vi "Main.vi"(10 "acqpanel":refnum<vi>, 11 "Module Admin":refnum<class "Delacor_lib_QMH_Module Admin.lvclass">) -> ()   [LabVIEW 2019, in "Adquisiion2.lvlib"]
doc: "This template is based off of the Queued Message Handler design pattern and the Queued Message Handler project template that ships with LabVIEW.\n\nThe main difference is that the queue is private to this module and communication between modules is performed via Broadcast and Request events.\n\nRequest events are wrapped in public API methods and are handled in the Event Handling Loop (EHL) of this VI. Any module can register for Broadcast events sent by this module. The EHL generates messages based on user interface actions.\n\nThe Message Handling Loop (MHL) processes messages generated by the EHL, or by other messages. The messages are string values, so new messages can be added easily to the Message Cases case structure in the MHL. Each message cluster can also provide an optional value for Message Data, which is a variant that can be converted to whatever message-specific data is required.\n_____\nBased on Delacor QMH Project Template 5.0.0.82."
uses:
  Adquisiion2.lvlib
  <vilib>/Delacor/Delacor QMH/Libraries/Module Admin_class/Delacor_lib_QMH_Module Admin.lvclass
  Module Data--cluster.ctl
  stop helper loop Argument--cluster.ctl
  <vilib>/Delacor/Delacor QMH/Libraries/Message Queue_class/Delacor_lib_QMH_Message Queue.lvclass/Delacor_lib_QMH_Message Queue.ctl
  Stop Argument--cluster.ctl
  <vilib>/Delacor/Delacor QMH/Libraries/Module Admin_class/Delacor_lib_QMH_Module Admin.lvclass/Delacor_lib_QMH_Module Admin.ctl
  <vilib>/Utility/miscctls.llb/LVPointTypeDef.ctl
  <vilib>/Delacor/Delacor QMH/Libraries/Message Queue_class/Delacor_lib_QMH_Enqueue Message (Single).vi
  <vilib>/Delacor/Delacor QMH/Libraries/Module Admin_class/Delacor_lib_QMH_Get External Launch.vi
  <vilib>/Utility/error.llb/Error Cluster From Error Code.vi
  <vilib>/ErrorRing/Error Ring.xnode
  <vilib>/Delacor/Delacor QMH/Libraries/Message Queue_class/Delacor_lib_QMH_Message Queue.lvclass
panel:
  out "Time Stamp":timestamp
  in  "Simulate MHL Error":bool
  in  "Simulate EHL Error":bool
  out "error out":errorcluster
  out "Status":string
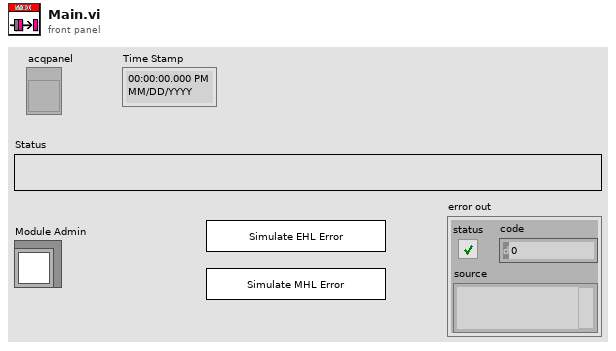
[diagram p1: front panel]
types:
  T1 = typedef "Adquisiion2.lvlib/Request Events--cluster.ctl" = cluster{"Stop Module":refnum<user-event>, "Show Panel":refnum<user-event>, "Hide Panel":refnum<user-event>, "Get Module Execution Status":refnum<user-event>, "Show Diagram":refnum<user-event>, "Start helper loop":refnum<user-event>, "stop helper loop":refnum<user-event>}
  T2 = typedef "Adquisiion2.lvlib/Module Data--cluster.ctl" = cluster{"Status":string}
  T3 = typedef "Adquisiion2.lvlib/stop helper loop Argument--cluster.ctl" = cluster{"Boolean":bool}
  T4 = enum32{"invalid lock state", "Not Locked", "Locked (No Password)", "Password-protected"}
  T5 = typedef "Adquisiion2.lvlib/Stop Argument--cluster.ctl" = cluster{"Origin":string, "Exit via Stop Module Req?":bool, "Wait for Module to stop?":bool}
  T6 = typedef "LVPointTypeDef.ctl" = cluster{"Horizontal":i16, "Vertical":i16}
  T7 = enum32{"Invalid", "Standard", "Closed", "Hidden", "Minimized", "Maximized"}
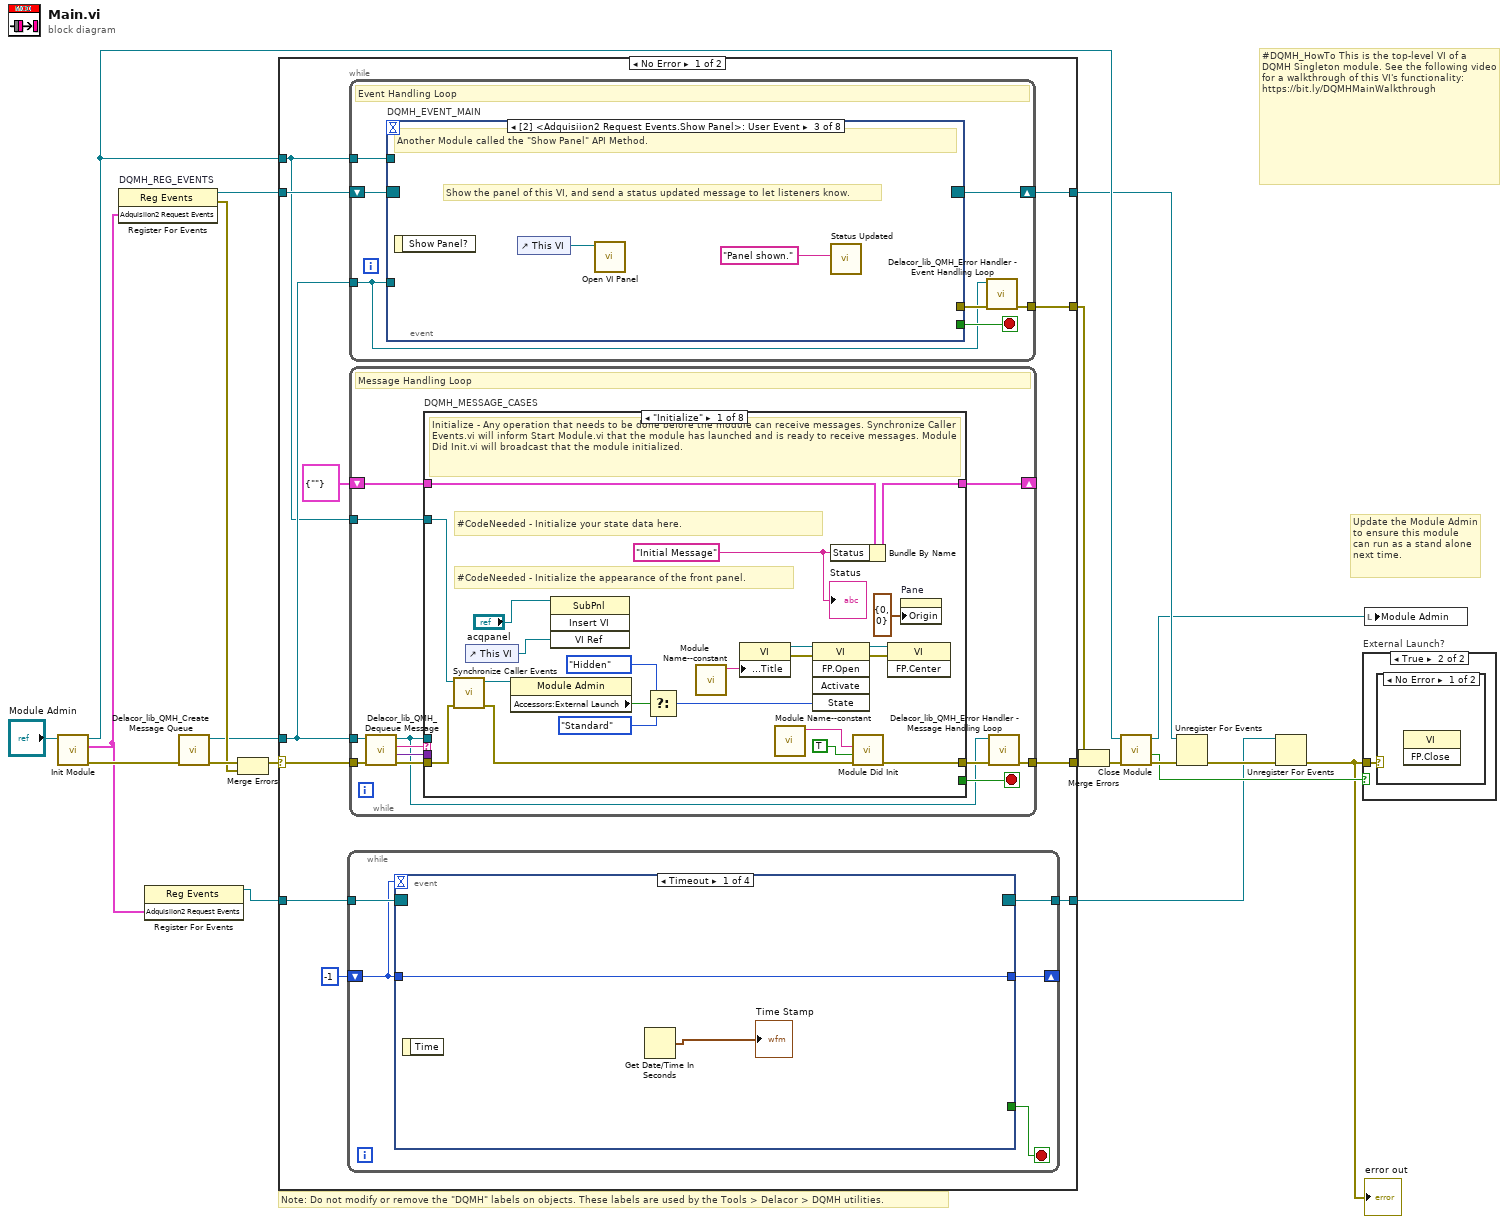
[diagram p0: block diagram]
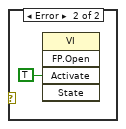
[diagram p3: hidden frame]
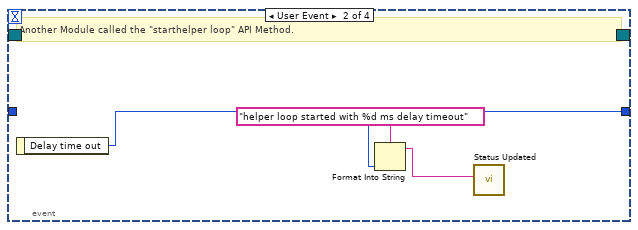
[diagram p4: hidden frame]
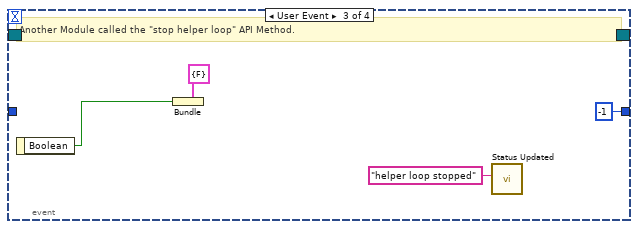
[diagram p5: hidden frame]
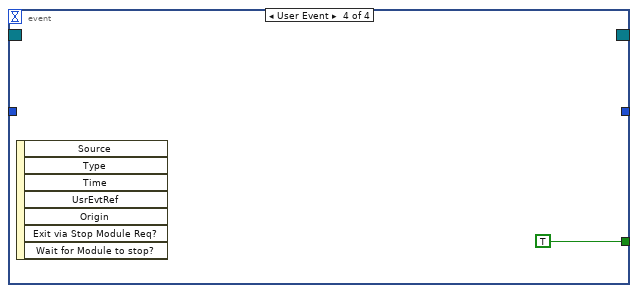
[diagram p6: hidden frame]
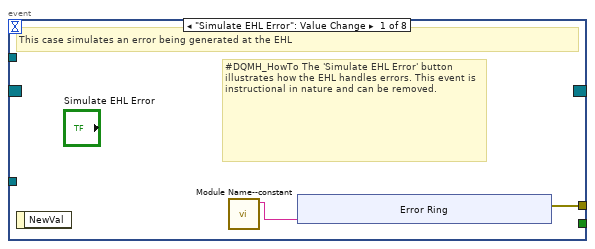
[diagram p7: hidden frame]
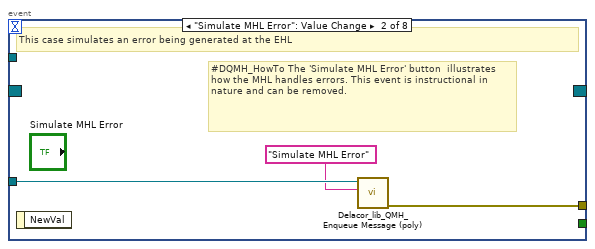
[diagram p8: hidden frame]
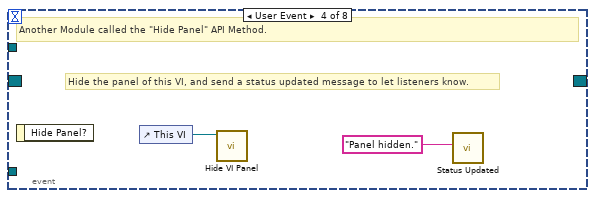
[diagram p9: hidden frame]
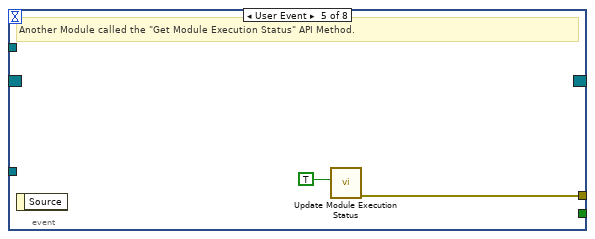
[diagram p10: hidden frame]
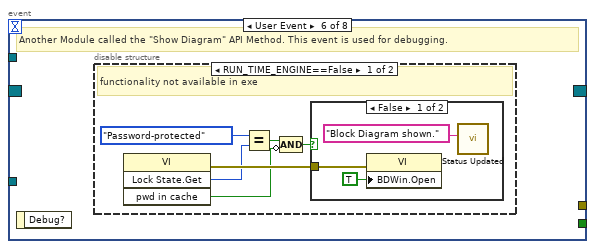
[diagram p11: hidden frame]
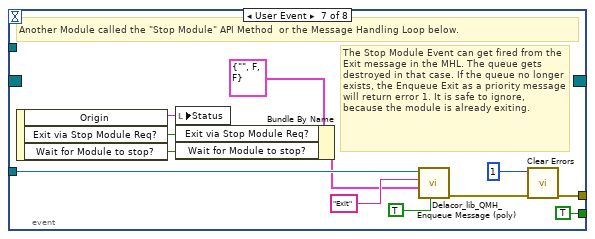
[diagram p14: hidden frame]
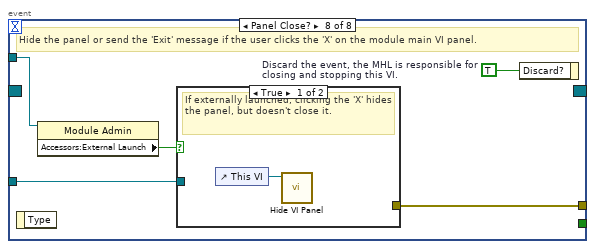
[diagram p15: hidden frame]
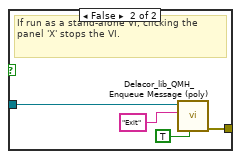
[diagram p16: hidden frame]
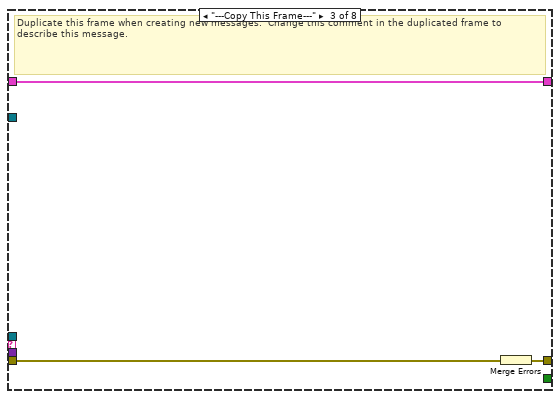
[diagram p18: hidden frame]
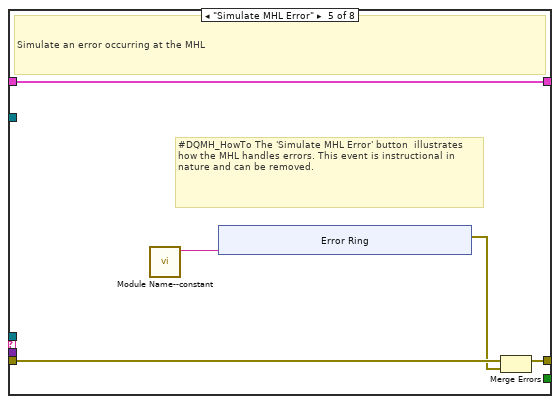
[diagram p20: hidden frame]
diagram:
  # "#DQMH_HowTo This is the top-level VI of a DQMH Singleton module. See the following video for a walkthrough of this VI's functionality: https://bit.ly/DQMHMainWalkthrough"
  # "Note: Do not modify or remove the \"DQMH\" labels on objects. These labels are used by the Tools > Delacor > DQMH utilities."
  # "Update the Module Admin to ensure this module can run as a stand alone next time."
  n1 = call "Init Module.vi"("Singleton Module Admin in"="Module Admin") -> ("error out"=w19:errorcluster, "Adquisiion2 Request Events"=w4:T1, "Singleton Module Admin out"=w12:refnum<class "Delacor_lib_QMH_Module Admin.lvclass">)  [unwired: 8 in]
  n2 = register-events "DQMH_REG_EVENTS"(w4) -> (reference out=w10:refnum<event-registration>, error out=w13:errorcluster)  [unwired: 2 in]
  n3 = register-events(w4) -> (reference out=w5:refnum<event-registration>)  [unwired: 2 in, 1 out]
  n4 = call <vilib>:"Delacor_lib_QMH_Create Message Queue.vi"("error in (no error)"=w19) -> ("error out"=w15:errorcluster, "Message Queue"=w9:refnum<class "Delacor_lib_QMH_Message Queue.lvclass">)  [unwired: 9 in]
  n5 = Merge Errors(w15, w13) -> (w14:errorcluster)
  n6 = case shown="No Error" w14 {
    selector: w14 -> [w29 w205]
    tunnel: [w31 w204] -> w20
    tunnel: [w28 w210] -> w11
    tunnel: w10 -> [w26 w210]
    tunnel: w9 -> [w25 w203]
    tunnel: [w30 _] -> w17
    tunnel: w12 -> [w24 w206]
    tunnel: w5 -> [w23 w202]
    tunnel: [w22 w202] -> w1
    frame No Error {
      n7 = while {
        tunnel: w23 -> [w36]
        tunnel: [w35] -> w22
        shift-right: [w33] -> _
        shift-left: -1 -> [w32]
        stop <- w34 stop-if-true
        n8 = event shown="[0] Timeout" {
          selector: w36 -> [_ _ _ _]
          dyn-events: [_ _ _ _] -> w35
          timeout: w32 -> [_ _ _ _]
          tunnel: [_ _ _ TRUE] -> w34
          tunnel: [w38 w41 -1 _] -> w33
          tunnel: w32 -> [w38 _ _ _]
          event Timeout {
            n9 = event-data() -> ()  [unwired: 1 in, 1 out]
            n10 = Get Date/Time In Seconds() -> (seconds since 1Jan1904=→"Time Stamp":timestamp)
          }
          event User Event {
            # "Another Module called the \"starthelper loop\" API Method."
            n11 = event-data() -> ("Delay time out"=w41:i32)  [unwired: 1 in]
            n12 = Format Into String(format string="helper loop started with %d ms delay timeout", w41) -> (resulting string=w40:string)  [unwired: 2 in, 1 out]
            n13 = call "Status Updated.vi"("Status"=w40) -> ()  [unwired: 10 in, 1 out]
          }
          event User Event {
            # "Another Module called the \"stop helper loop\" API Method."
            n14 = event-data() -> ("Boolean"=w44:bool)  [unwired: 1 in]
            n15 = Bundle(cluster=T3 {"Boolean"=FALSE} ("stop helper loop Argument"), "Boolean"=w44) -> ()  [unwired: 1 out]
            n16 = call "Status Updated.vi"("Status"="helper loop stopped") -> ()  [unwired: 10 in, 1 out]
          }
          event User Event {
            n17 = event-data() -> ()  [unwired: 1 in, 7 out]
          }
        }
      }
      n18 = while {
        tunnel: w25 -> [w47]
        shift-right: [w50] -> w28
        shift-left: w26 -> [w51]
        tunnel: [w52] -> w30
        tunnel: w24 -> [w48]
        stop <- w49 stop-if-true
        # "Event Handling Loop"
        n19 = event "DQMH_EVENT_MAIN" shown="[2] <Adquisiion2 Request Events.Show Panel>: User Event" {
          selector: w51 -> [_ _ _ _ _ _ _ _]
          dyn-events: [_ _ _ _ _ _ _ _] -> w50
          timeout: _ -> [_ _ _ _ _ _ _ _]
          tunnel: [_ _ _ _ _ _ TRUE ("Discard?") _] -> w49
          tunnel: w47 -> [_ w64 _ _ _ _ w88 w95]
          tunnel: [w55 w65 _ _ w71 _ w91 w97] -> w53
          tunnel: w48 -> [_ _ _ _ _ _ _ w94]
          event "Simulate EHL Error": Value Change {
            # "#DQMH_HowTo The 'Simulate EHL Error' button  illustrates how the EHL handles errors. This event is instructional in nature and can be removed."
            # "This case simulates an error being generated at the EHL"
            n20 = event-data() -> ()  [unwired: 1 in, 1 out]
            n21 = call "Module Name--constant.vi"() -> ("Module Name"=w54:string)  [unwired: 11 in]
            n22 = xnode "Error Ring"("parameter 0"=w54) -> ("error out"=w55:errorcluster)
          }
          event "Simulate MHL Error": Value Change {
            # "#DQMH_HowTo The 'Simulate MHL Error' button  illustrates how the MHL handles errors. This event is instructional in nature and can be removed."
            # "This case simulates an error being generated at the EHL"
            n23 = event-data() -> ()  [unwired: 1 in, 1 out]
            n24 = call-poly <vilib>:"Delacor_lib_QMH_Enqueue Message (poly).vi"("Message"="Simulate MHL Error", "Message Queue in"=w64) -> ("error out"=w65:errorcluster)  [unwired: 8 in, 1 out]
          }
          event User Event {
            # "Show the panel of this VI, and send a status updated message to let listeners know."
            # "Another Module called the \"Show Panel\" API Method."
            n25 = event-data() -> ()  [unwired: 1 in, 1 out]
            n26 = control-ref of="This VI"() -> (w67:refnum<vi>)
            n27 = call "Open VI Panel.vi"("VI"=w67) -> ()  [unwired: 10 in, 1 out]
            n28 = call "Status Updated.vi"("Status"="Panel shown." ("format string")) -> ()  [unwired: 10 in, 1 out]
          }
          event User Event {
            # "Hide the panel of this VI, and send a status updated message to let listeners know."
            # "Another Module called the \"Hide Panel\" API Method."
            n29 = event-data() -> ()  [unwired: 1 in, 1 out]
            n30 = control-ref of="This VI"() -> (w69:refnum<vi>)
            n31 = call "Hide VI Panel.vi"("VI"=w69) -> ()  [unwired: 10 in, 1 out]
            n32 = call "Status Updated.vi"("Status"="Panel hidden." ("format string")) -> ()  [unwired: 10 in, 1 out]
          }
          event User Event {
            # "Another Module called the \"Get Module Execution Status\" API Method."
            n33 = event-data() -> ()  [unwired: 1 in, 1 out]
            n34 = call "Update Module Execution Status.vi"("Running?"=TRUE) -> ("error out"=w71:errorcluster)  [unwired: 10 in]
          }
          event User Event {
            # "Another Module called the \"Show Diagram\" API Method. This event is used for debugging."
            n35 = event-data() -> ()  [unwired: 1 in, 1 out]
            n36 = disable-structure shown="RUN_TIME_ENGINE==False" {
              frame condition #0 (active) {
                # "functionality not available in exe"
                n37 = invoke class="VI" method="Lock State.Get"() -> (error out=w77:errorcluster, "Get Lock State"=w76:T4, "pwd in cache"=w73:bool)  [unwired: 4 in, 1 out]
                n38 = Equal?(x=T4."Password-protected", y=w76) -> (x = y?=w74:bool)
                n39 = Compound Arithmetic op=AND(w74, invert w73) -> (w72:bool)
                n40 = case shown="False" w72 {
                  tunnel: w77 -> [w80 _]
                  frame False {
                    n41 = property class="VI"(error in=w80, "BDWin.Open"=TRUE ("Block Diagram Window:Open")) -> ()  [unwired: 1 in, 2 out]
                    n42 = call "Status Updated.vi"("Status"="Block Diagram shown." ("format string")) -> ()  [unwired: 10 in, 1 out]
                  }
                  frame True {
                    # "Password-protected VI, and the password is not in the cache. Do not show the diagram."
                  }
                }
              }
              frame condition #1 {
              }
            }
          }
          event User Event {
            # "The Stop Module Event can get fired from the Exit message in the MHL. The queue gets destroyed in that case. If the queue no longer exists, the Enqueue Exit as a priority message will return error 1. It is safe to ignore, because the module is already exiting."
            # "Another Module called the \"Stop Module\" API Method  or the Message Handling Loop below."
            n43 = event-data() -> ("Origin"=w87:string, "Exit via Stop Module Req?"=w83:bool, "Wait for Module to stop?"=w82:bool)  [unwired: 1 in]
            n44 = local write "Status"(w87) -> ()
            n45 = Bundle By Name(cluster=T5 {"Origin"="", "Exit via Stop Module Req?"=FALSE, "Wait for Module to stop?"=FALSE} ("Stop Argument"), "Exit via Stop Module Req?"=w83, "Wait for Module to stop?"=w82) -> (w81:T5)
            n46 = call-poly <vilib>:"Delacor_lib_QMH_Enqueue Message (poly).vi"("Priority Message? (F)"=TRUE, "Message Data"=w81, "Message"="Exit", "Message Queue in"=w88) -> ("error out"=w92:errorcluster)  [unwired: 6 in, 1 out]
            n47 = call <vilib>:"Clear Errors.vi"("error in (no error)"=w92, "specific error code to clear (0: all)"=1) -> ("error out"=w91:errorcluster)  [unwired: 4 in, 1 out]
          }
          event Panel Close? {
            w96 = TRUE  # Discard the event, the MHL is responsible for closing and stopping this VI.
            # "Hide the panel or send the 'Exit' message if the user clicks the 'X' on the module main VI panel."
            n48 = event-data() -> ()  [unwired: 1 in, 1 out]
            n49 = property class="Module Admin"(reference=w94) -> ("Accessors:External Launch"=w93:bool)  [unwired: 1 in, 2 out]
            n50 = case shown="True" w93 {
              tunnel: w95 -> [_ w101]
              tunnel: [_ w102] -> w97
              frame True {
                # "If externally launched, clicking the 'X' hides the panel, but doesn't close it."
                n51 = control-ref of="This VI"() -> (w98:refnum<vi>)
                n52 = call "Hide VI Panel.vi"("VI"=w98) -> ()  [unwired: 10 in, 1 out]
              }
              frame False {
                # "If run as a stand-alone VI, clicking the panel 'X' stops the VI."
                n53 = call-poly <vilib>:"Delacor_lib_QMH_Enqueue Message (poly).vi"("Priority Message? (F)"=TRUE, "Message"="Exit", "Message Queue in"=w101) -> ("error out"=w102:errorcluster)  [unwired: 7 in, 1 out]
              }
            }
            n54 = event-data("Discard?"=w96) -> ()  [unwired: 1 in, 1 out]
          }
        }
        n55 = call-dynamic "Delacor_lib_QMH_Error Handler - Event Handling Loop.vi"("error in (no error)"=w53, "Message Queue in"=w47) -> ("dup error in"=w52:errorcluster)  [unwired: 8 in, 1 out]
      }
      n56 = while {
        tunnel: w25 -> [w105]
        shift-right: [w109] -> _
        shift-left: T2 {"Status"=""} ("Data Cluster") -> [w110]
        tunnel: w29 -> [w113]
        tunnel: [w111] -> w31
        tunnel: w24 -> [w103]
        stop <- w108 stop-if-true
        # "Message Handling Loop"
        n57 = call-dynamic "Delacor_lib_QMH_Dequeue Message.vi"("error in (no error)"=w113, "Message Queue in"=w105) -> ("error out"=w112:errorcluster, "Message Data"=w106:variant, "Message"=w107:string, "Message Queue out"=w104:refnum<class "Delacor_lib_QMH_Message Queue.lvclass">)  [unwired: 6 in]
        n58 = case "DQMH_MESSAGE_CASES" shown="\"Initialize\"" w107 {
          selector: w107 -> [_ _ _ _ _ _ _ w189]
          tunnel: w104 -> [_ _ _ _ _ w159 w181 _]
          tunnel: w112 -> [w134 w138 w141 w143 w148 w166 w187 w191]
          tunnel: [w132 w138 w140 w143 w147 w162 w184 w192] -> w114
          tunnel: w110 -> [w123 w137 w139 w142 w145 w161 w180 w190]
          tunnel: [w122 w137 w139 w142 w145 w161 w180 w190] -> w109
          tunnel: [_ _ _ _ _ _ w179 _] -> w108
          tunnel: w106 -> [_ _ _ _ _ w160 w178 _]
          tunnel: w103 -> [w124 _ _ _ _ w158 w173 _]
          frame "Initialize" {
            w117 = "Initial Message" ("Initial Message")
            # "#CodeNeeded - Initialize the appearance of the front panel."
            # "#CodeNeeded - Initialize your state data here."
            # "Initialize - Any operation that needs to be done before the module can receive messages. Synchronize Caller Events.vi will inform Start Module.vi that the module has launched and is ready to receive messages. Module Did Init.vi will broadcast that the module initialized."
            n59 = call "Synchronize Caller Events.vi"("error in (no error)"=w134, "Singleton Module Admin in"=w124) -> ("error out"=w133:errorcluster, "Singleton Module Admin out"=w119:refnum<class "Delacor_lib_QMH_Module Admin.lvclass">)  [unwired: 8 in]
            n60 = control-ref of="This VI"() -> (w115:refnum<vi>)
            n61 = property class="Module Admin"(reference=w119) -> ("Accessors:External Launch"=w128:bool)  [unwired: 1 in, 2 out]
            n62 = invoke class="SubPnl" method="Insert VI"(reference="acqpanel", "VI Ref"=w115) -> ()  [unwired: 2 in, 4 out]
            n63 = Select(t=T7."Hidden" ("State"), s=w128, f=T7."Standard" ("State")) -> (s? t:f=w125:T7)
            n64 = call "Module Name--constant.vi"() -> ("Module Name"=w131:string)  [unwired: 11 in]
            n65 = property class="VI"("Front Panel.Title"=w131) -> (reference out=w130:refnum<vi>, error out=w136:errorcluster)  [unwired: 2 in]
            n66 = call "Module Name--constant.vi"() -> ("Module Name"=w120:string)  [unwired: 11 in]
            n67 = invoke class="VI" method="FP.Open"(reference=w130, error in=w136, "State"=w125) -> (reference out=w129:refnum<vi>, error out=w135:errorcluster)  [unwired: 2 in, 3 out]
            n68 = Bundle By Name(cluster=w123, "Status"=w117) -> (w122:T2)
            n69 = call "Module Did Init.vi"("error in (no error)"=w133, "Initialized?"=TRUE, "Origin"=w120) -> ("error out"=w132:errorcluster)  [unwired: 8 in]
            n70 = invoke class="VI" method="FP.Center"(reference=w129, error in=w135) -> ()  [unwired: 1 in, 3 out]
            n71 = property on="Pane" class="Pane"("Origin"=T6 {"Horizontal"=0, "Vertical"=0}) -> ()  [unwired: 2 in, 2 out]
            "Status" <- w117
          }
          frame "--- Module Specific ---" {
            # "Separator -- The following cases handle messages specific to this Module."
          }
          frame "---Copy This Frame---" {
            # "Duplicate this frame when creating new messages.  Change this comment in the duplicated frame to describe this message."
            n72 = Merge Errors(w141) -> (w140:errorcluster)
          }
          frame "--- Exit and Error Handling---" {
            # "Separator - The following cases handle errors and exit messages."
          }
          frame "Simulate MHL Error" {
            # "#DQMH_HowTo The 'Simulate MHL Error' button  illustrates how the MHL handles errors. This event is instructional in nature and can be removed."
            # "Simulate an error occurring at the MHL"
            n73 = call "Module Name--constant.vi"() -> ("Module Name"=w144:string)  [unwired: 11 in]
            n74 = xnode "Error Ring"("parameter 0"=w144) -> ("error out"=w146:errorcluster)
            n75 = Merge Errors(w148, w146) -> (w147:errorcluster)
          }
          frame "Error" {
            # "#CodeRecommended - If you ever change the name of this \"Error\" message, you'll need to update the name in the Check Loop Error.vi as well."
            # "#CodeRecommended - If the module is running in standalone mode (External Launch = FALSE), this code will pop up an error dialog and call the 'Exit' message if an error occurs. Add more fine-grained error handling here."
            # "Error - Check the error message data and respond accordingly. This message is sent by the \"Error Handler\" VIs at the end of each loop in this application."
            n76 = property class="Module Admin"(reference=w158) -> ("Accessors:External Launch"=w157:bool)  [unwired: 1 in, 2 out]
            n77 = Variant To Data(error in=w166, type=errorcluster {"status"=FALSE, "code"=0, "source"=""} ("error constant"), Variant=w160) -> (data=w167:errorcluster, error out=w164:errorcluster)
            n78 = call "Module Name--constant.vi"() -> ("Module Name"=w156:string)  [unwired: 11 in]
            n79 = call "Error Reported.vi"("Additional Information"=w156, "Error"=w167) -> ()  [unwired: 9 in, 1 out]
            n80 = case shown="False" w157 {
              tunnel: [w172 _] -> w163
              tunnel: w159 -> [w170 _]
              tunnel: w167 -> [w171 _]
              frame False {
                # "If the module is running standalone, then pop up an error dialog and call the \"Exit\" message."
                n81 = call <vilib>:"Simple Error Handler.vi"("error in (no error)"=w171) -> ()  [unwired: 4 in, 5 out]
                n82 = call-poly <vilib>:"Delacor_lib_QMH_Enqueue Message (poly).vi"("Priority Message? (F)"=TRUE, "Message"="Exit", "Message Queue in"=w170) -> ("error out"=w172:errorcluster)  [unwired: 7 in, 1 out]
              }
              frame True {
                # "If the module was launched externally, calling the Error Reported broadcast VI is the only action performed by the \"Error\" message. The module's caller can then process the error appropriately."
              }
            }
            n83 = Merge Errors(w164, w163) -> (w162:errorcluster)
            n84 = local write "error out"(w162) -> ()
          }
          frame "Exit" {
            w177 = 91  # 91: not all Exit messages will have an argument
            w179 = TRUE  # Stop the VI
            # "Release the message queue reference"
            # "#CodeNeeded - Add any required cleanup code here"
            # "Exit - Exit the application."
            n85 = Variant To Data(error in=w187, type=T5 {"Origin"="", "Exit via Stop Module Req?"=FALSE, "Wait for Module to stop?"=FALSE} ("Stop Argument"), Variant=w178) -> (data=w175:T5, error out=w183:errorcluster)
            n86 = call <vilib>:"Clear Errors.vi"("error in (no error)"=w183, "specific error code to clear (0: all)"=w177) -> ("error out"=w186:errorcluster)  [unwired: 4 in, 1 out]
            n87 = control-ref of="This VI"() -> (w174:refnum<vi>)
            n88 = call-dynamic "Delacor_lib_QMH_Release Message Queue.vi"("error in (no error)"=w186, "Message Queue"=w181) -> ("error out"=w185:errorcluster)  [unwired: 9 in]
            n89 = call "Handle Exit.vi"("Stop Argument"=w175, "Admin in"=w173, "VI reference"=w174) -> ("error out"=w182:errorcluster)  [unwired: 7 in, 1 out]
            n90 = Merge Errors(w185, w182) -> (w184:errorcluster)
          }
          frame Default {
            # "'Default' case only runs if there is a message that isn't defined in any of the other cases.  Output a programming error."
            n91 = call "Module Name--constant.vi"() -> ("Module Name"=w188:string)  [unwired: 11 in]
            n92 = xnode "Error Ring"("parameter 0"=w189, "parameter 1"=w188) -> ("error out"=w193:errorcluster)
            n93 = Merge Errors(w191, w193) -> (w192:errorcluster)
          }
        }
        n94 = call-dynamic "Delacor_lib_QMH_Error Handler - Message Handling Loop.vi"("error in (no error)"=w114, "Message Queue in"=w104) -> ("dup error in"=w111:errorcluster)  [unwired: 8 in, 1 out]
      }
    }
    frame Error {
      # "Synchronize Caller Events.vi will inform Start Module.vi that the module has launched and will let the code calling Start Module.vi register for broadcasts and would permit the caller receive the broadcast that an error occurred at launch time."
      n95 = call-dynamic "Delacor_lib_QMH_Release Message Queue.vi"("error in (no error)"=w205, "Message Queue"=w203) -> ("error out"=w204:errorcluster)  [unwired: 9 in]
      n96 = call "Synchronize Caller Events.vi"("Singleton Module Admin in"=w206) -> ("error out"=w211:errorcluster)  [unwired: 9 in, 1 out]
      n97 = call "Module Name--constant.vi"() -> ("Module Name"=w209:string)  [unwired: 11 in]
      n98 = Format Into String(format string="An error occurred during initialization. %s is no longer running.", w209) -> (resulting string=w207:string)  [unwired: 2 in, 1 out]
      n99 = Merge Errors(w204, w211) -> (w212:errorcluster)
      n100 = call "Error Reported.vi"("Additional Information"=w207, "Error"=w212) -> ()  [unwired: 9 in, 1 out]
    }
  }
  n101 = Merge Errors(w17, w20) -> (w16:errorcluster)
  n102 = call "Close Module.vi"("error in (no error)"=w16, "Module Admin in"=w12) -> ("error out"=w18:errorcluster, "External Launch"=w6:bool, "Module Admin out"=w7:refnum<class "Delacor_lib_QMH_Module Admin.lvclass">)  [unwired: 7 in]
  n103 = Unregister For Events(event registration refnum=w11, error in=w18) -> (error out=w3:errorcluster)
  n104 = Unregister For Events(event registration refnum=w1, error in=w3) -> (error out=w2:errorcluster)
  "error out" <- w2
  n105 = case "External Launch?" shown="True" w6 {
    tunnel: w2 -> [_ w213]
    frame False {
    }
    frame True {
      n106 = case shown="No Error" w213 {
        frame No Error {
          n107 = invoke class="VI" method="FP.Close"() -> ()  [unwired: 3 in, 3 out]
        }
        frame Error {
          n108 = invoke class="VI" method="FP.Open"("Activate"=TRUE ("Activate?")) -> ()  [unwired: 4 in, 5 out]
        }
      }
    }
  }
  n109 = local write "Module Admin"(w7) -> ()
